vi "Update Graph.vi"(8 "error in (no error)":errorcluster, 11 "Controller in":refnum<class "Controller.lvclass">) -> (0 "error out":errorcluster, 3 "Controller out":refnum<class "Controller.lvclass">)   [LabVIEW 2019, in "Controller.lvlib" / "Controller.lvclass"]
uses:
  Controller.lvclass
  Counts.ctl
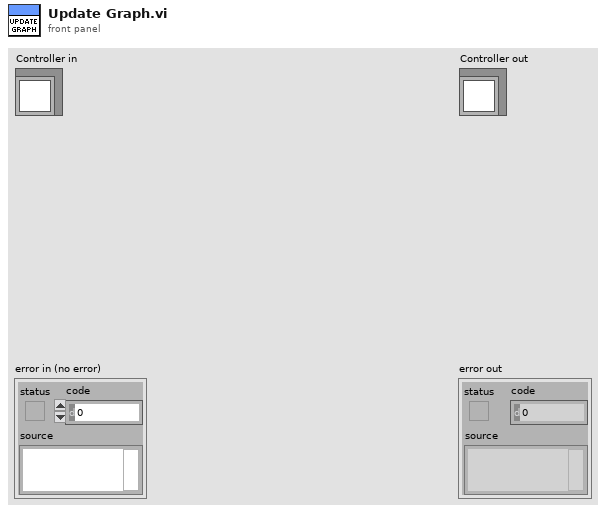
[diagram p1: front panel]
types:
  T1 = typedef "Counts.ctl" = cluster{"Single Master Events":i32, "Single Slave Events":i32, "Coincident Events":i32, "Single Master Event Rate":dbl, "Single Slave Event Rate":dbl, "Coincident Event Rate":dbl}
  T2 = cluster{"Single Master Events":i32, "Single Slave Events":i32, "Coincident Events":i32}
  T3 = typedef "Muon Detector.lvclass/Event.ctl" = cluster{"Event Count":i32, "Device Timestamp (ms)":i32, "PC Timestamp":timestamp, "ADC Count":i32, "Event Type":u8}
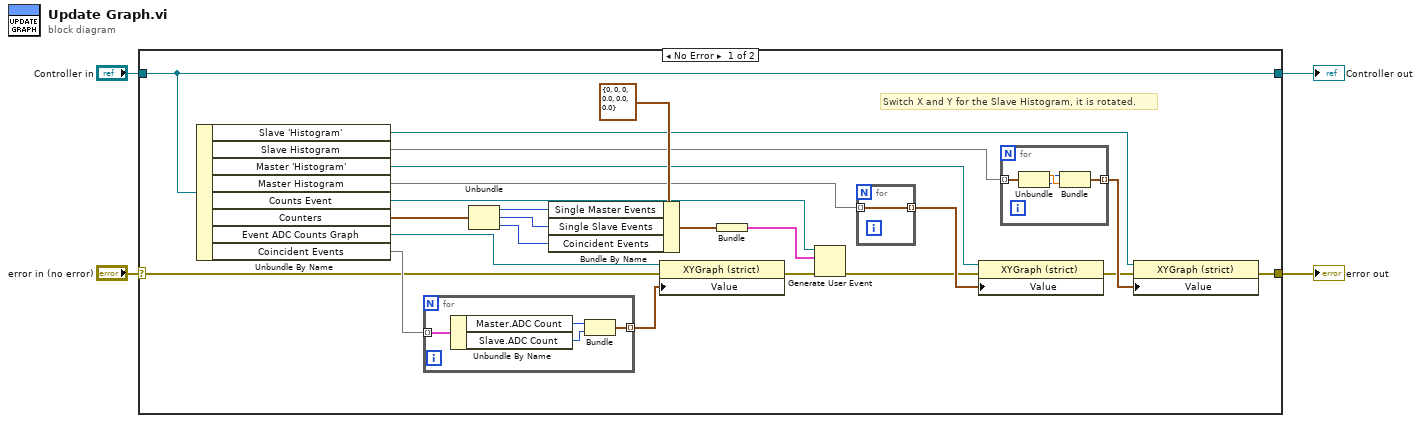
[diagram p0: block diagram]
diagram:
  n1 = case shown="No Error" "error in (no error)" {
    selector: "error in (no error)" -> [w23 w38]
    tunnel: [w10 w38] -> w3
    tunnel: [w27 w37] -> w1
    tunnel: "Controller in" -> [w27 w37]
    frame No Error {
      # "Switch X and Y for the Slave Histogram, it is rotated."
      n2 = Unbundle By Name(w27) -> ("Slave 'Histogram'"=w12:refnum<vi>, "Slave Histogram"=w14:map{dbl, i32}, "Master 'Histogram'"=w17:refnum<vi>, "Master Histogram"=w16:map{dbl, i32}, "Counts Event"=w9:refnum<user-event>, "Counters"=w21:T2, "Event ADC Counts Graph"=w25:refnum<vi>, "Coincident Events"=w26:set{cluster{"Master":T3, "Slave":T3}})
      n3 = for {
        tunnel: w26 -> [w36] mode=indexing
        tunnel: [w33] -> w24 mode=indexing
        n4 = Unbundle By Name(w36) -> ("Master.ADC Count"=w35:i32, "Slave.ADC Count"=w34:i32)
        n5 = Bundle("ADC Count"=w35, "ADC Count"=w34) -> (w33:cluster{"ADC Count":i32, "ADC Count":i32})  [unwired: 1 in]
      }
      n6 = Unbundle(w21) -> ("Single Master Events"=w20:i32, "Single Slave Events"=w19:i32, "Coincident Events"=w18:i32)
      n7 = Bundle By Name(cluster=T1 {"Single Master Events"=0, "Single Slave Events"=0, "Coincident Events"=0, "Single Master Event Rate"=0.0, "Single Slave Event Rate"=0.0, "Coincident Event Rate"=0.0} ("Value"), "Single Master Events"=w20, "Single Slave Events"=w19, "Coincident Events"=w18) -> (w6:T1)
      n8 = property class="XYGraph (strict)"(reference=w25, error in=w23, "Value"=w24) -> (error out=w8:errorcluster)  [unwired: 1 out]
      n9 = Bundle("Value"=w6) -> (w5:cluster{"Value":T1})  [unwired: 1 in]
      n10 = Generate User Event(user event=w9, event data cluster=w5, error in=w8) -> (error out=w7:errorcluster)  [unwired: 1 in, 1 out]
      n11 = for {
        tunnel: w16 -> [w32] mode=indexing
        tunnel: [w32] -> w15 mode=indexing
      }
      n12 = property class="XYGraph (strict)"(reference=w17, error in=w7, "Value"=w15) -> (error out=w11:errorcluster)  [unwired: 1 out]
      n13 = for {
        tunnel: w14 -> [w31] mode=indexing
        tunnel: [w30] -> w13 mode=indexing
        n14 = Unbundle(w31) -> (w29:dbl, w28:i32)
        n15 = Bundle(w28, w29) -> (w30:cluster{i32, dbl})  [unwired: 1 in]
      }
      n16 = property class="XYGraph (strict)"(reference=w12, error in=w11, "Value"=w13) -> (error out=w10:errorcluster)  [unwired: 1 out]
    }
    frame Error {
    }
  }
  "error out" <- w3
  "Controller out" <- w1
